vi "VoltageShift.vi"(9 "Cutoff":dbl=11.0 format="%#_13g", 10 "Current Voltage":dbl, 11 "Shift Input":T1=enum."Reverse") -> (3 "Shift Output":T1)   [LabVIEW 2017]
uses:
  <vilib>/Rock Robotics/WPI/Solenoid/WPI_SolenoidValue.ctl
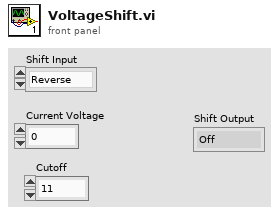
[diagram p1: front panel]
types:
  T1 = typedef "WPI_SolenoidValue.ctl" = enum16{"Off", "On", "Forward", "Reverse"}
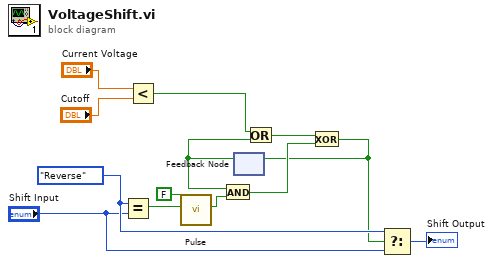
[diagram p0: block diagram]
diagram:
  w13 = WPI_SolenoidValue."Reverse" ("Shift Value")
  n1 = Equal?(x=w13, y="Shift Input") -> (x = y?=w7:bool)
  n2 = Less?(x="Current Voltage", y="Cutoff") -> (x < y?=w10:bool)
  n3 = call "Pulse.vi"("Input"=w7, "Rising Edge?"=FALSE) -> ("Output"=w9:bool)  [unwired: 9 in]
  n4 = feedback #1() -> (w11:bool)  [unwired: 1 in]
  n5 = And(x=w11, y=w9) -> (x .and. y?=w2:bool)
  n6 = Or(x=w10, y=w11) -> (x .or. y?=w3:bool)
  n7 = Exclusive Or(1:w2, 2:w3) -> (0:w1:bool)
  n8 = feedback-in #1(w1) -> ()
  n9 = Select(t=w13, s=w1, f="Shift Input") -> (s? t:f=→"Shift Output":T1)
